vi "Configure Acquisition Record Core.vi"(0 "CS++Scope":refnum<class "CS++Scope.lvclass">, 5 "time per record (1.0E-3 s)":dbl[unit]=0.001 format="%^.2e", 7 "min record length (100 samples)":i32=100, 9 "acquisition start time (0.0 s)":dbl[unit] format="%.3f", 11 "error in (no error)":errorcluster) -> (4 "CS++Scope out":refnum<class "CS++Scope.lvclass">, 15 "error out":errorcluster)   [LabVIEW 2016, in "CS++Scope.lvlib" / "CS++Scope.lvclass"]
doc: "This VI configures the most commonly configured properties of the oscilloscope acquisition subsystem. These properties are the time per record, minimum record length, and the acquisition start time."
uses:
  CS++Scope.lvclass
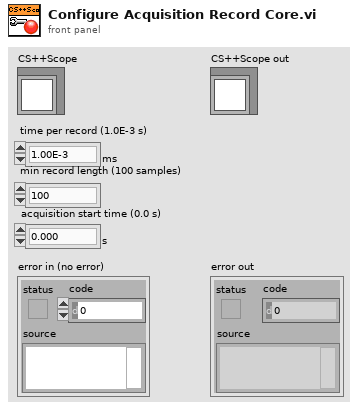
[diagram p1: front panel]
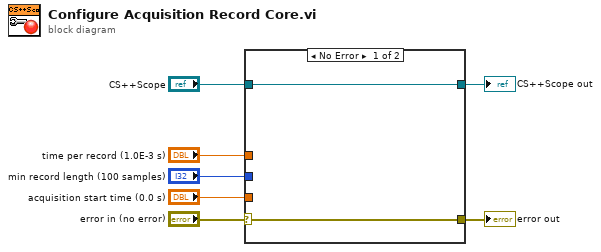
[diagram p0: block diagram]
diagram:
  n1 = case shown="No Error" "error in (no error)" {
    selector: "error in (no error)" -> [w8 w11]
    tunnel: [w8 w11] -> w6
    tunnel: [w9 w10] -> w2
    tunnel: "CS++Scope" -> [w9 w10]
    tunnel: "time per record (1.0E-3 s)" -> [_ _]
    tunnel: "min record length (100 samples)" -> [_ _]
    tunnel: "acquisition start time (0.0 s)" -> [_ _]
    frame No Error {
    }
    frame Error {
    }
  }
  "error out" <- w6
  "CS++Scope out" <- w2
